vi "Main.vi"() -> ()   [LabVIEW 2018]
uses:
  Framework/CntrlRefs.ctl
  Modules/BusClass/Bus.lvclass/Bus.ctl
  LV_Config_class/Config.lvclass/Config.ctl
  Modules/Sync/SyncModule/PublicAPI/Arguments/Broadcasts/clDidInit.ctl
  <userlib>/NIST/ModuleAdminLib/ModuleAdmin/ModuleAdmin.lvclass
  LV_Config_class/Typedefs/eLogLvl.ctl
  Framework/UserEvents/clUserEventDataType.ctl
  LV_TestAutomation/Comms_lib/CommsData.ctl
  Modules/BusClass/Accessors/Read BusNumber.vi
  Modules/BusClass/Accessors/Read Test.vi
  LV_Config_class/Accessors/Read Root Directory.vi
  Modules/BusClass/Accessors/Write Test.vi
  LV_Config_class/Accessors/Read ConfigFilePath.vi
  <extravilib>/ChannelInstances/Tag-bool/Read With Abort.vi
  <extravilib>/ChannelInstances/Tag-bool/Write With Abort.vi
  <vilib>/Utility/error.llb/Error Cluster From Error Code.vi
  <extravilib>/ChannelInstances/Tag-bool/Instantiate.vi
  <extravilib>/ChannelInstances/Tag-bool/EndpointRead.vi
  <extravilib>/ChannelInstances/Tag-bool/Endpoint.vi
  <vilib>/ErrorRing/Error Ring.xnode
  Modules/TestClass/Test.lvclass
  Framework/Queue/Queue.lvlib
  <userlib>/NIST/NISTErrorLib/NISTErrorLib.lvlib
  LV_Config_class/Config.lvclass
  LV_Ini/Ini_lib.lvlib
  <vilib>/Utility/config.llb/NI_LVConfig.lvlib
  Modules/BusClass/Bus.lvclass
  Modules/Sync/SyncModule/SyncModule.lvlib
  Modules/FGen/FgenModule/FgenModule.lvlib
  Modules/Digitizer/DigitizerModule/DigitizerModule.lvlib
  Modules/Analysis/AnalysisModule/AnalysisModule.lvlib
  Modules/Sensor/SensorModule/SensorModule.lvlib
  Modules/Visualization/Visualization.lvlib
  LV_TestAutomation/LV-PY_Lib/LV-PY.lvlib
  LV_TestAutomation/Comms_lib/Comms.lvlib
  <extravilib>/ChannelInstances/Tag-bool.lvlib
panel:
  in  "btnAbort":bool
  in  "btnSettings":bool
  in  "btnHideMods":bool caption="Hide Modules"
  in  "chkLeaveScriptWindowOpen":bool
  in  "btnScriptFile":bool
  in  "Test Script":string
  in  "btnVisualize":bool
  out "Locked":bool
  in  "btnSyncPref":bool
  in  "rngSync":u16(ring) caption="Sync" items=["Local", "NI PXI 6682", "Debug Sync IOP", "6683H class Dyn3", "AbsPhase", "CorrFactor", "Debug", "SaveWaveform", "Dyn3 PMU Cal", "HIL_Sync", "INRM", "Legacy", "Offset Digi Trigger", "PXI Multi"]
  in  "btnSensorPref":bool
  in  "rngSensor":u16(ring) caption="Sensor" items=["C37.118 PMU", "C37.118 Sim", "Base PMU", "none", "Sim Ideal PMU"]
  in  "btnRunOne":bool
  in  "btnRunScript":bool
  in  "btnAnalysisPref":bool
  in  "rngAnalysis":u16(ring) caption="Analysis" items=["None", "AbsPhase", "FFT", "INRIM_Comp", "PMU", "AbsPhase_1M", "Analyse Waveforms"]
  in  "btnDigitizerPref":bool
  in  "rngDigitizer":u16(ring) caption="Digitizer" items=["Agilent3458", "IVI Digitizer", "AbsPhase_Current", "AbsPhase_Voltage", "Analyse Waveforms", "Debug", "INRiM_3Ch", "INRiM_4Ch", "INRiM_5Ch", "INRiM_6Ch", "INRM_1Ch", "Offset Trigger", "PMU Cal", "PRS_FGen", "Simulation"]
  in  "btnFGenPref":bool
  in  "rngFGen":u16(ring) caption="Function Generator" items=["DaqMx_Single", "Single_AM", "None", "Agilent IVI FGen", "IVI Dual FGens", "IVI FGen", "AbsPhase_Current_1Phase_ao3", "AbsPhase_Current_5A_ao0", "AbsPhase_Voltage_10V_Direct", "AbsPhase_Voltage_70V_Amp", "Debug", "INRM_1Ch", "INRM", "Pxi6733_Sine", "Pxi6733 Sine Standalone", "PMU Cal", "PMU_Sim", "Test"]
  in  "btnTestFile":bool
  in  "Test File":string
  in  "btnStop":bool
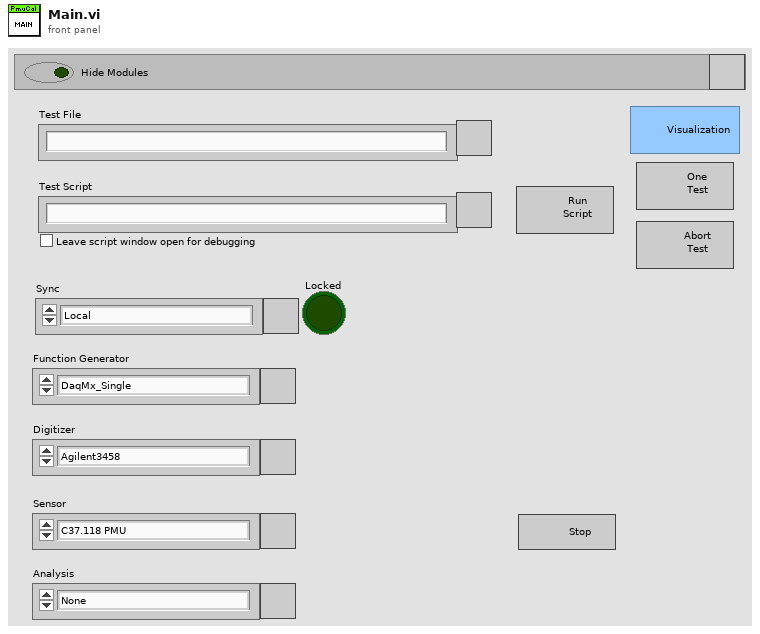
[diagram p1: front panel]
types:
  T1 = typedef "CntrlRefs.ctl" = cluster{"rngFGen":refnum<vi>, "rngDigitizer":refnum<vi>, "rngAnalysis":refnum<vi>, "rngSync":refnum<vi>, "btnHideMods":refnum<vi>, "rngSensor":refnum<vi>, "Test Script":refnum<vi>}
  T2 = typedef "SyncModule.lvlib/clBroadcastEvents.ctl" = cluster{"DidInit":refnum<user-event>, "StatusUpdate":refnum<user-event>, "ErrorReport":refnum<user-event>, "DidStop":refnum<user-event>, "PathToINI":refnum<user-event>, "TriggerTime":refnum<user-event>, "LockStatus":refnum<user-event>, "Info":refnum<user-event>, "ClockProperties":refnum<user-event>}
  T3 = typedef "FgenModule.lvlib/clBroadcastEvents.ctl" = cluster{"DidInit":refnum<user-event>, "StatusUpdate":refnum<user-event>, "ErrorReport":refnum<user-event>, "DidStop":refnum<user-event>, "PathToINI":refnum<user-event>, "Channels":refnum<user-event>, "Function":refnum<user-event>, "Waveforms":refnum<user-event>, "Triggers":refnum<user-event>, "FunctionParams":refnum<user-event>, "FunctionArbs":refnum<user-event>, "FunctionSampleRate":refnum<user-event>}
  T4 = typedef "DigitizerModule.lvlib/clBroadcastEvents.ctl" = cluster{"DidInit":refnum<user-event>, "StatusUpdate":refnum<user-event>, "ErrorReport":refnum<user-event>, "DidStop":refnum<user-event>, "PathToINI":refnum<user-event>, "Channels":refnum<user-event>, "Acq":refnum<user-event>, "Trigger":refnum<user-event>, "Waveforms":refnum<user-event>}
  T5 = typedef "SensorShared.lvlib/clBroadcastEvents.ctl" = cluster{"DidInit":refnum<user-event>, "StatusUpdate":refnum<user-event>, "ErrorReport":refnum<user-event>, "DidStop":refnum<user-event>, "PathToINI":refnum<user-event>, "SensorReport":refnum<user-event>, "SensorConfig":refnum<user-event>}
  T6 = typedef "AnalysisModule.lvlib/clBroadcastEvents.ctl" = cluster{"DidInit":refnum<user-event>, "StatusUpdate":refnum<user-event>, "ErrorReport":refnum<user-event>, "DidStop":refnum<user-event>, "PathToINI":refnum<user-event>, "Config":refnum<user-event>, "ResultReport":refnum<user-event>, "FunctionClass":refnum<user-event>, "State":refnum<user-event>, "FunctionParams":refnum<user-event>}
  T7 = typedef "clUserEvents.ctl" = cluster{"StopEvent":refnum<user-event>, "CreateBus":refnum<user-event>, "UpdateEvents":refnum<user-event>}
  T8 = typedef "clUserEventDataType.ctl" = cluster{"Data":variant}
  T9 = typedef "Comms.lvlib/CommsData.ctl" = cluster{"Command":string, "XMLData":string}
  T10 = typedef "NI_LVConfig.lvlib/Config Data RefNum.ctl" = refnum<k1>
  T11 = typedef "Config_class.lvlib/Config.lvclass/RootDir.ctl" = cluster{"pathRootDir":path, "btnOutPath":bool, "OutDir":string, "btnOpenOutputDir":bool, "ScriptDir":string, "btnOpenScriptDir":bool, "TestDir":string, "btnOpenTestDir":bool}
  T12 = typedef "Tag-bool.lvlib/))Channel.ctl" = refnum<queue>
  T13 = typedef "Config_class.lvlib/Config.lvclass/eLogLvl.ctl" = enum16{"Normal", "Verbose", "None"}
  T14 = typedef "SyncModule.lvlib/clDidInit.ctl" = cluster{"Init?":bool, "ModuleAdmin":refnum<class "ModuleAdmin.lvclass">}
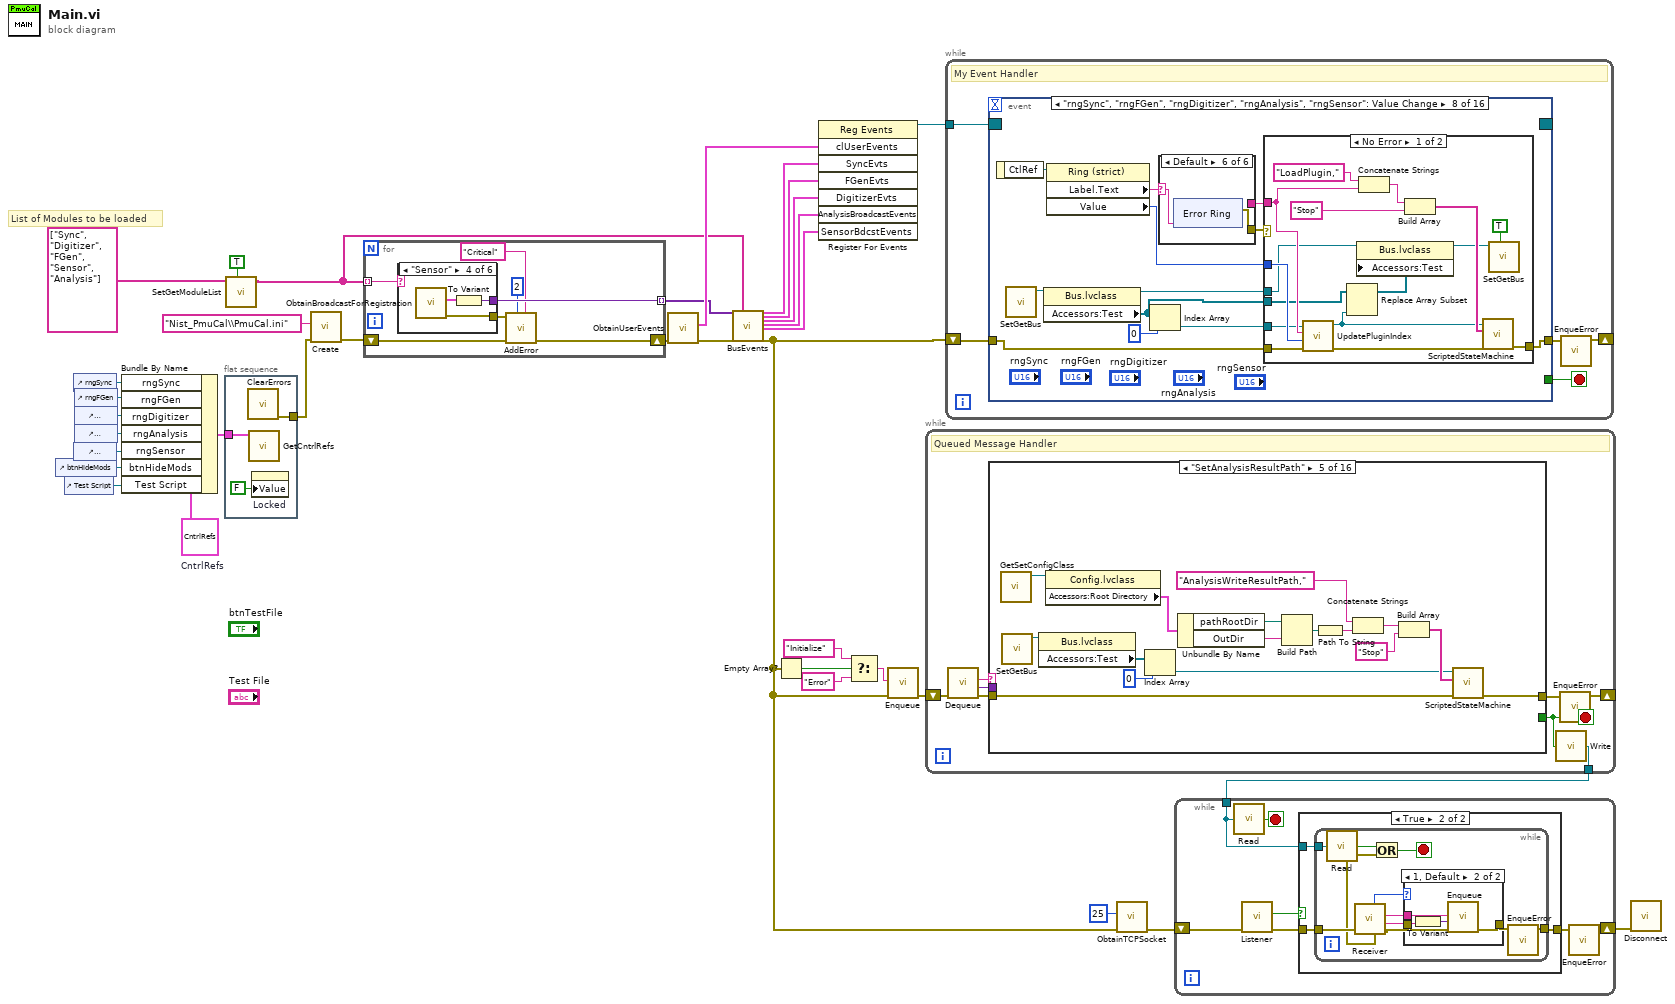
[diagram p0: block diagram]
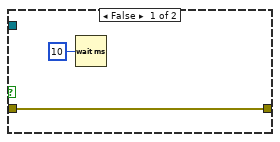
[diagram p2: hidden frame]
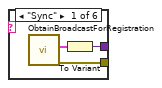
[diagram p4: hidden frame]
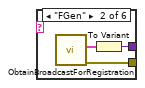
[diagram p5: hidden frame]
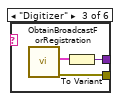
[diagram p6: hidden frame]
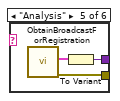
[diagram p7: hidden frame]
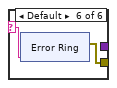
[diagram p8: hidden frame]
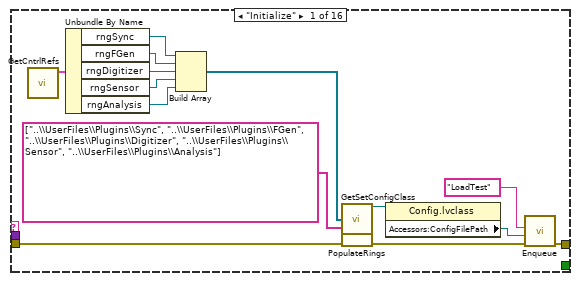
[diagram p9: hidden frame]
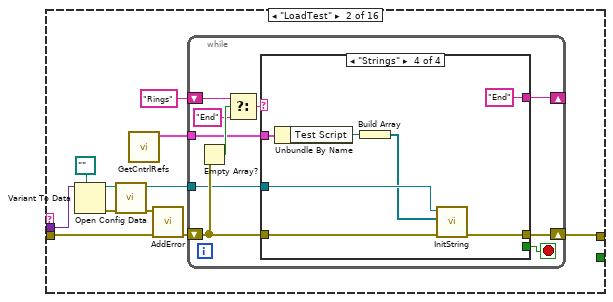
[diagram p10: hidden frame]
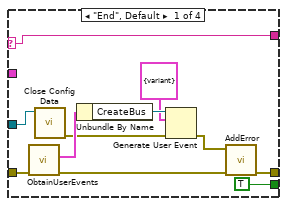
[diagram p11: hidden frame]
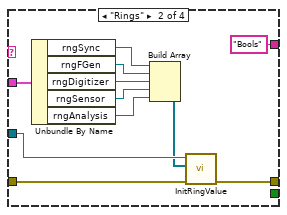
[diagram p12: hidden frame]
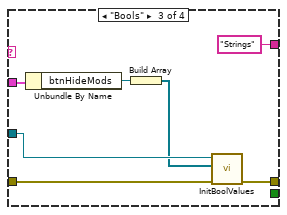
[diagram p13: hidden frame]
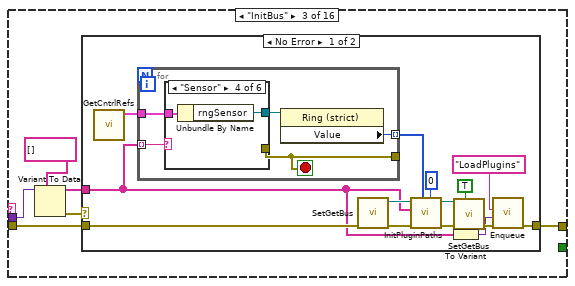
[diagram p14: hidden frame]
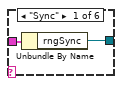
[diagram p15: hidden frame]
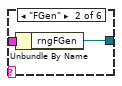
[diagram p16: hidden frame]
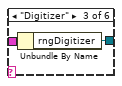
[diagram p17: hidden frame]
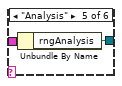
[diagram p18: hidden frame]
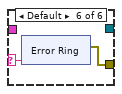
[diagram p19: hidden frame]
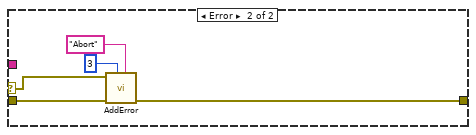
[diagram p20: hidden frame]
diagram:
  w31 = T1 {"rngFGen"=refnum, "rngDigitizer"=refnum, "rngAnalysis"=refnum, "rngSync"=refnum, "btnHideMods"=refnum, "rngSensor"=refnum, "Test Script"=refnum}  # CntrlRefs
  # "List of Modules to be loaded"
  n1 = control-ref of="btnHideMods"() -> (w9:refnum<vi>)
  n2 = control-ref of="Test Script"() -> (w2:refnum<vi>)
  n3 = control-ref of="rngSync"() -> (w23:refnum<vi>)
  n4 = control-ref of="rngSensor"() -> (w8:refnum<vi>)
  n5 = control-ref of="rngFGen"() -> (w30:refnum<vi>)
  n6 = control-ref of="rngDigitizer"() -> (w28:refnum<vi>)
  n7 = control-ref of="rngAnalysis"() -> (w27:refnum<vi>)
  n8 = Bundle By Name(cluster=w31, "rngSync"=w23, "rngFGen"=w30, "rngDigitizer"=w28, "rngAnalysis"=w27, "rngSensor"=w8, "btnHideMods"=w9, "Test Script"=w2) -> (w29:T1)
  n9 = flat-sequence {
    tunnel: [w38] -> w32
    tunnel: w29 -> [w37]
    frame #0 {
      n10 = call <userlib>:"ClearErrors.vi"() -> ("ErrorArray"=w38:errorcluster[])  [unwired: 11 in]
      n11 = call "GetCntrlRefs.vi"("CntrlRefs"=w37) -> ()  [unwired: 10 in, 1 out]
      n12 = property on="Locked" class="Bool (strict)"("Value"=FALSE) -> ()  [unwired: 2 in, 2 out]
    }
  }
  n13 = call "SetGetModuleList.vi"("Set? (f)"=TRUE, "ModuleList"=string[] ["Sync", "Digitizer", "FGen", "Sensor", "Analysis"]) -> ("ModuleList"=w12:string[])  [unwired: 9 in]
  n14 = call "Create.vi"("ErrorArray"=w32, "name or relative path"="Nist_PmuCal\\PmuCal.ini") -> ("ErrorArray"=w18:errorcluster[])  [unwired: 8 in, 1 out]
  n15 = for {
    shift-right: [w44] -> w17
    shift-left: w18 -> [w43]
    tunnel: [w42] -> w14 mode=indexing
    tunnel: w12 -> [w39] mode=indexing
    n16 = case shown="\"Sensor\"" w39 {
      selector: w39 -> [_ _ _ _ _ w61]
      tunnel: [w47 w50 w53 w56 w59 _] -> w42
      tunnel: [w46 w51 w54 w57 w60 w62] -> w45
      frame "Sync" {
        n17 = call "ObtainBroadcastForRegistration.vi"() -> ("error out"=w46:errorcluster, "SyncBroadcastEvents"=w48:T2)  [unwired: 10 in]
        n18 = To Variant(anything=w48) -> (Variant=w47:variant)
      }
      frame "FGen" {
        n19 = call "ObtainBroadcastForRegistration.vi"() -> ("error out"=w51:errorcluster, "clBroadcastEvents"=w49:T3)  [unwired: 10 in]
        n20 = To Variant(anything=w49) -> (Variant=w50:variant)
      }
      frame "Digitizer" {
        n21 = call "ObtainBroadcastForRegistration.vi"() -> ("error out"=w54:errorcluster, "clDigitizerBdcstEvents"=w52:T4)  [unwired: 10 in]
        n22 = To Variant(anything=w52) -> (Variant=w53:variant)
      }
      frame "Sensor" {
        n23 = call "ObtainBroadcastForRegistration.vi"() -> ("error out"=w57:errorcluster, "SensorBdcstEvents"=w55:T5)  [unwired: 10 in]
        n24 = To Variant(anything=w55) -> (Variant=w56:variant)
      }
      frame "Analysis" {
        n25 = call "ObtainBroadcastForRegistration.vi"() -> ("error out"=w60:errorcluster, "AnalysisBroadcastEvents"=w58:T6)  [unwired: 10 in]
        n26 = To Variant(anything=w58) -> (Variant=w59:variant)
      }
      frame Default {
        n27 = xnode "Error Ring"("parameter 0"=w61) -> ("error out"=w62:errorcluster)
      }
    }
    n28 = call <userlib>:"AddError.vi"("Severity"="Critical", "Priority"=u8 2, "ErrorArray"=w43, "error in (no error)"=w45) -> ("ErrorArray"=w44:errorcluster[])  [unwired: 6 in, 1 out]
  }
  n29 = call "ObtainUserEvents.vi"("ErrorArray"=w17) -> ("ErrorArray"=w16:errorcluster[], "clUserEvents"=w15:T7)  [unwired: 9 in]
  n30 = call "BusEvents.vi"("EventArray"=w14, "Error in"=w16, "ModuleList"=w12) -> ("SyncEvts"=w26:T2, "FGenEvts"=w25:T3, "DigitizerEvts"=w24:T4, "AnalysisBroadcastEvents"=w10:T6, "SensorBdcstEvents"=w7:T5, "Error out"=w6:errorcluster[])  [unwired: 16 in, 3 out]
  n31 = Empty Array?(array=w6) -> (empty?=w22:bool)
  n32 = register-events(w15, w26, w25, w24, w10, w7) -> (reference out=w35:refnum<event-registration>)  [unwired: 2 in, 1 out]
  n33 = Select(t="Initialize" ("Message"), s=w22, f="Error" ("Message")) -> (s? t:f=w19:string)
  n34 = call "Enqueue.vi"("ErrorArray"=w6, "Message"=w19) -> ("ErrorArray"=w34:errorcluster[])  [unwired: 9 in]
  n35 = while {
    shift-right: [w74] -> _
    shift-left: w34 -> [w77]
    tunnel: [w70] -> w1
    stop <- w71 stop-if-true
    # "Queued Message Handler"
    n36 = call "Dequeue.vi"("ErrorArray"=w77) -> ("ErrorArray"=w73:errorcluster[], "Message Data"=w72:variant, "Message"=w76:string)  [unwired: 8 in]
    n37 = case shown="\"SetAnalysisResultPath\"" w76 {
      selector: w76 -> [_ _ _ _ _ _ _ _ _ _ _ _ _ _ _ w415]
      tunnel: [w90 w93 w151 w198 w222 w240 w296 w306 w329 w349 w356 w366 w372 w375 w388 w413] -> w75
      tunnel: w73 -> [w86 w98 w152 w199 w228 w246 w301 w320 w333 w353 w360 w367 w374 w376 _ w412]
      tunnel: [_ _ _ _ _ _ _ _ _ _ _ _ _ TRUE _ _] -> w71
      tunnel: w72 -> [_ w97 w154 w201 _ w248 _ _ w335 w355 w364 _ _ _ w392 _]
      frame "Initialize" {
        n38 = call "GetCntrlRefs.vi"() -> ("CntrlRefs"=w85:T1)  [unwired: 11 in]
        n39 = Unbundle By Name(w85) -> ("rngSync"=w79:refnum<vi>, "rngFGen"=w84:refnum<vi>, "rngDigitizer"=w83:refnum<vi>, "rngSensor"=w82:refnum<vi>, "rngAnalysis"=w78:refnum<vi>)
        n40 = Build Array(w79, w84, w83, w82, w78) -> (w80:refnum<vi>[])
        n41 = call "GetSetConfigClass.vi"() -> ("Ref out"=w91:refnum<class "Config.lvclass">)  [unwired: 11 in]
        n42 = call "PopulateRings.vi"("ErrorArray In"=w86, "RelativePathToIniArray"=string[] ["..\\UserFiles\\Plugins\\Sync", "..\\UserFiles\\Plugins\\FGen", "..\\UserFiles\\Plugins\\Digitizer", "..\\UserFiles\\Plugins\\Sensor", "..\\UserFiles\\Plugins\\Analysis"], "RingRefArray"=w80) -> ("ErrorArray Out"=w87:errorcluster[])  [unwired: 7 in, 1 out]
        n43 = property class="Config.lvclass"(reference=w91) -> ("Accessors:ConfigFilePath"=w89:path)  [unwired: 1 in, 2 out]
        n44 = call "Enqueue.vi"("ErrorArray"=w87, "Message Data"=w89, "Message"="LoadTest") -> ("ErrorArray"=w90:errorcluster[])  [unwired: 8 in]
      }
      frame "LoadTest" {
        n45 = Variant To Data(type=path "", Variant=w97) -> (data=w101:path, error out=w99:errorcluster)  [unwired: 1 in]
        n46 = call <vilib>:"Open Config Data.vi"("error in (no error)"=w99, "configuration file path"=w101) -> ("error out"=w100:errorcluster, "refnum"=w95:T10)  [unwired: 7 in, 1 out]
        n47 = call "GetCntrlRefs.vi"() -> ("CntrlRefs"=w92:T1)  [unwired: 11 in]
        n48 = call <userlib>:"AddError.vi"("ErrorArray"=w98, "error in (no error)"=w100) -> ("ErrorArray"=w96:errorcluster[])  [unwired: 8 in, 1 out]
        n49 = while {
          shift-right: [w106] -> w93
          shift-left: w96 -> [w108]
          tunnel: w95 -> [w107]
          shift-right: [w104] -> _
          shift-left: "Rings" -> [w111]
          tunnel: w92 -> [w103]
          stop <- w105 stop-if-true
          n50 = Empty Array?(array=w108) -> (empty?=w112:bool)
          n51 = Select(t=w111, s=w112, f="End") -> (s? t:f=w109:string)
          n52 = case shown="\"Strings\"" w109 {
            selector: w109 -> [w120 _ _ _]
            tunnel: w108 -> [w119 w134 w139 w147]
            tunnel: w107 -> [w123 w133 w137 w145]
            tunnel: [w122 w127 w138 w146] -> w106
            tunnel: [TRUE _ _ _] -> w105
            tunnel: [w120 "Bools" "Strings" "End"] -> w104
            tunnel: w103 -> [_ w126 w140 w144]
            frame "End", Default {
              n53 = call "ObtainUserEvents.vi"("ErrorArray"=w119) -> ("ErrorArray"=w113:errorcluster[], "clUserEvents"=w118:T7)  [unwired: 9 in]
              n54 = call <vilib>:"Close Config Data.vi"("refnum"=w123) -> ("error out"=w116:errorcluster)  [unwired: 9 in, 1 out]
              n55 = Unbundle By Name(w118) -> ("CreateBus"=w117:refnum<user-event>)
              n56 = Generate User Event(user event=w117, event data cluster=T8 {"Data"=variant} ("clUserEventData"), error in=w116) -> (error out=w114:errorcluster)  [unwired: 1 in, 1 out]
              n57 = call <userlib>:"AddError.vi"("ErrorArray"=w113, "error in (no error)"=w114) -> ("ErrorArray"=w122:errorcluster[])  [unwired: 8 in, 1 out]
            }
            frame "Rings" {
              n58 = Unbundle By Name(w126) -> ("rngSync"=w125:refnum<vi>, "rngFGen"=w130:refnum<vi>, "rngDigitizer"=w131:refnum<vi>, "rngSensor"=w129:refnum<vi>, "rngAnalysis"=w124:refnum<vi>)
              n59 = Build Array(w125, w130, w131, w129, w124) -> (w128:refnum<vi>[])
              n60 = call "InitRingValue.vi"("ErrorArray In"=w134, "RingRefArray"=w128, "IniFileRef"=w133) -> ("ErrorArray Out"=w127:errorcluster[])  [unwired: 6 in, 2 out]
            }
            frame "Bools" {
              n61 = Unbundle By Name(w140) -> ("btnHideMods"=w136:refnum<vi>)
              n62 = Build Array(w136) -> (w135:refnum<vi>[])
              n63 = call "InitBoolValues.vi"("ErrorArray in"=w139, "BoolRefArray"=w135, "IniFileRef in"=w137) -> ("ErrorArray Out"=w138:errorcluster[])  [unwired: 7 in, 1 out]
            }
            frame "Strings" {
              n64 = Unbundle By Name(w144) -> ("Test Script"=w143:refnum<vi>)
              n65 = Build Array(w143) -> (w142:refnum<vi>[])
              n66 = call "InitString.vi"("ErrorArray in"=w147, "StringRefArray"=w142, "IniFileRef in"=w145) -> ("ErrorArray Out"=w146:errorcluster[])  [unwired: 7 in, 1 out]
            }
          }
        }
      }
      frame "InitBus" {
        n67 = Variant To Data(type=string[] [], Variant=w154) -> (data=w150:string[], error out=w149:errorcluster)  [unwired: 1 in]
        n68 = case shown="No Error" w149 {
          selector: w149 -> [_ w193]
          tunnel: w152 -> [w166 w195]
          tunnel: [w158 w194] -> w151
          tunnel: w150 -> [w155 _]
          frame No Error {
            n69 = call "GetCntrlRefs.vi"() -> ("CntrlRefs"=w165:T1)  [unwired: 11 in]
            n70 = for {
              tunnel: w155 -> [w171] mode=indexing
              tunnel: w165 -> [w170]
              tunnel: [w168] -> w163 mode=indexing
              tunnel: [w167] -> _
              stop <- w167 stop-if-true
              n71 = case shown="\"Sensor\"" w171 {
                selector: w171 -> [_ _ _ _ _ w183]
                tunnel: w170 -> [w173 w175 w177 w179 w181 _]
                tunnel: [w172 w174 w176 w178 w180 _] -> w169
                tunnel: [_ _ _ _ _ w182] -> w167
                frame "Sync" {
                  n72 = Unbundle By Name(w173) -> ("rngSync"=w172:refnum<vi>)
                }
                frame "FGen" {
                  n73 = Unbundle By Name(w175) -> ("rngFGen"=w174:refnum<vi>)
                }
                frame "Digitizer" {
                  n74 = Unbundle By Name(w177) -> ("rngDigitizer"=w176:refnum<vi>)
                }
                frame "Sensor" {
                  n75 = Unbundle By Name(w179) -> ("rngSensor"=w178:refnum<vi>)
                }
                frame "Analysis" {
                  n76 = Unbundle By Name(w181) -> ("rngAnalysis"=w180:refnum<vi>)
                }
                frame Default {
                  n77 = xnode "Error Ring"("parameter 0"=w183) -> ("error out"=w182:errorcluster)
                }
              }
              n78 = property class="Ring (strict)"(reference=w169) -> ("Value"=w168:u16)  [unwired: 1 in, 2 out]
            }
            n79 = call "SetGetBus.vi"() -> ("Bus.lvclass"=w164:refnum<class "Bus.lvclass">)  [unwired: 11 in]
            n80 = call "InitPluginPaths.vi"("BusIndex"=0, "PluginIndex"=w163, "Error In"=w166, "Modules"=w155, "Bus in"=w164) -> ("Error Out"=w159:errorcluster[], "Bus out"=w161:refnum<class "Bus.lvclass">)  [unwired: 5 in]
            n81 = To Variant(anything=w155) -> (Variant=w156:variant)
            n82 = call "SetGetBus.vi"("Set (f)"=TRUE, "Bus.lvclass"=w161) -> ()  [unwired: 9 in, 1 out]
            n83 = call "Enqueue.vi"("ErrorArray"=w159, "Message Data"=w156, "Message"="LoadPlugins") -> ("ErrorArray"=w158:errorcluster[])  [unwired: 8 in]
          }
          frame Error {
            n84 = call <userlib>:"AddError.vi"("Severity"="Abort", "Priority"=u8 3, "ErrorArray"=w195, "error in (no error)"=w193) -> ("ErrorArray"=w194:errorcluster[])  [unwired: 6 in, 1 out]
          }
        }
      }
      frame "LoadPlugins" {
        n85 = Variant To Data(type=string[] [], Variant=w201) -> (data=w197:string[], error out=w196:errorcluster)  [unwired: 1 in]
        n86 = case shown="No Error" w196 {
          selector: w196 -> [_ w219]
          tunnel: w199 -> [w210 w221]
          tunnel: [w203 w220] -> w198
          tunnel: w197 -> [w213 _]
          frame No Error {
            n87 = for {
              tunnel: w213 -> [w215] mode=indexing
              tunnel: [w214] -> w212 mode=indexing
              n88 = Concatenate Strings("LoadPlugin," ("string"), w215) -> (w214:string)
            }
            n89 = call "SetGetBus.vi"() -> ("Bus.lvclass"=w209:refnum<class "Bus.lvclass">)  [unwired: 11 in]
            n90 = property class="Bus.lvclass"(reference=w209) -> ("Accessors:Test"=w208:refnum<class "Test.lvclass">[])  [unwired: 1 in, 2 out]
            n91 = Index Array(array=w208, index=0) -> (element=w206:refnum<class "Test.lvclass">)
            n92 = Build Array (concatenate)(w212, "Stop" ("string")) -> (w205:string[])
            n93 = call "ScriptedStateMachine.vi"("ErrorArray"=w210, "script"=w205, "Test.lvclass"=w206) -> ("ErrorArray"=w204:errorcluster[])  [unwired: 6 in, 2 out]
            n94 = call "Enqueue.vi"("ErrorArray"=w204, "Message"="SetAnalysisResultPath") -> ("ErrorArray"=w203:errorcluster[])  [unwired: 9 in]
          }
          frame Error {
            n95 = call <userlib>:"AddError.vi"("Severity"="Abort", "Priority"=u8 3, "ErrorArray"=w221, "error in (no error)"=w219) -> ("ErrorArray"=w220:errorcluster[])  [unwired: 6 in, 1 out]
          }
        }
      }
      frame "SetAnalysisResultPath" {
        n96 = call "GetSetConfigClass.vi"() -> ("Ref out"=w237:refnum<class "Config.lvclass">)  [unwired: 11 in]
        n97 = call "SetGetBus.vi"() -> ("Bus.lvclass"=w226:refnum<class "Bus.lvclass">)  [unwired: 11 in]
        n98 = property class="Bus.lvclass"(reference=w226) -> ("Accessors:Test"=w225:refnum<class "Test.lvclass">[])  [unwired: 1 in, 2 out]
        n99 = property class="Config.lvclass"(reference=w237) -> ("Accessors:Root Directory"=w236:T11)  [unwired: 1 in, 2 out]
        n100 = Index Array(array=w225, index=0) -> (element=w223:refnum<class "Test.lvclass">)
        n101 = Unbundle By Name(w236) -> ("pathRootDir"=w235:path, "OutDir"=w234:string)
        n102 = Build Path(base path=w235, name or relative path=w234) -> (appended path=w233:path)
        n103 = Path To String(path=w233) -> (string=w232:string)
        n104 = Concatenate Strings("AnalysisWriteResultPath,", w232) -> (w230:string)
        n105 = Build Array(w230, "Stop") -> (w227:string[])
        n106 = call "ScriptedStateMachine.vi"("ErrorArray"=w228, "script"=w227, "Test.lvclass"=w223) -> ("ErrorArray"=w222:errorcluster[])  [unwired: 6 in, 2 out]
      }
      frame "SaveTest" {
        n107 = Variant To Data(type=path "", Variant=w248) -> (data=w244:path, error out=w239:errorcluster)  [unwired: 1 in]
        n108 = call <vilib>:"Open Config Data.vi"("error in (no error)"=w239, "configuration file path"=w244) -> ("error out"=w243:errorcluster, "refnum"=w242:T10)  [unwired: 7 in, 1 out]
        n109 = call "GetCntrlRefs.vi"() -> ("CntrlRefs"=w238:T1)  [unwired: 11 in]
        n110 = call <userlib>:"AddError.vi"("ErrorArray"=w246, "error in (no error)"=w243) -> ("ErrorArray"=w245:errorcluster[])  [unwired: 8 in, 1 out]
        n111 = while {
          tunnel: w242 -> [w258]
          shift-right: [w252] -> w240
          shift-left: w245 -> [w254]
          shift-right: [w250] -> _
          shift-left: "Rings" -> [w256]
          tunnel: w238 -> [w249]
          stop <- w251 stop-if-true
          n112 = Empty Array?(array=w254) -> (empty?=w255:bool)
          n113 = Select(t=w256, s=w255, f="end") -> (s? t:f=w257:string)
          n114 = case shown="\"Bools\"" w257 {
            selector: w257 -> [_ _ _ w284]
            tunnel: w254 -> [w266 w273 w283 w286]
            tunnel: w258 -> [w265 w272 w281 w289]
            tunnel: [w263 w270 w282 w285] -> w252
            tunnel: [_ _ _ TRUE] -> w251
            tunnel: ["Bools" "Strings" "End" w284] -> w250
            tunnel: w249 -> [w260 w275 w280 _]
            frame "Rings" {
              n115 = Unbundle By Name(w260) -> ("rngSync"=w261:refnum<vi>, "rngFGen"=w267:refnum<vi>, "rngDigitizer"=w269:refnum<vi>, "rngSensor"=w268:refnum<vi>, "rngAnalysis"=w259:refnum<vi>)
              n116 = Build Array(w261, w267, w269, w268, w259) -> (w264:refnum<vi>[])
              n117 = call "RingsToIni.vi"("ErrorArray in"=w266, "RingRefArray"=w264, "IniFileRef in"=w265) -> ("ErrorArray out"=w263:errorcluster[])  [unwired: 7 in, 1 out]
            }
            frame "Bools" {
              n118 = Unbundle By Name(w275) -> ("btnHideMods"=w274:refnum<vi>)
              n119 = Build Array(w274) -> (w271:refnum<vi>[])
              n120 = call "BoolsToIni.vi"("ErrorArray in"=w273, "BoolRefArray"=w271, "IniFileRef in"=w272) -> ("ErrorArray out"=w270:errorcluster[])  [unwired: 7 in, 1 out]
            }
            frame "Strings" {
              n121 = Unbundle By Name(w280) -> ("Test Script"=w279:refnum<vi>)
              n122 = Build Array(w279) -> (w278:refnum<vi>[])
              n123 = call "StringToIni.vi"("ErrorArray in"=w283, "StringRefArray"=w278, "IniFileRef in"=w281) -> ("ErrorArray out"=w282:errorcluster[])  [unwired: 7 in, 1 out]
            }
            frame "End", Default {
              n124 = call <vilib>:"Close Config Data.vi"("write file if changed (T)"=TRUE, "refnum"=w289) -> ("error out"=w287:errorcluster)  [unwired: 8 in, 1 out]
              n125 = call <userlib>:"AddError.vi"("ErrorArray"=w286, "error in (no error)"=w287) -> ("ErrorArray"=w285:errorcluster[])  [unwired: 8 in, 1 out]
            }
          }
        }
      }
      frame "RunOneTest" {
        n126 = call "SetGetModuleList.vi"() -> ("ModuleList"=w293:string[])  [unwired: 11 in]
        n127 = call "SetGetBus.vi"() -> ("Bus.lvclass"=w300:refnum<class "Bus.lvclass">)  [unwired: 11 in]
        n128 = for {
          tunnel: w293 -> [w303] mode=indexing
          shift-right: [w302] -> w294
          shift-left: "RunTest" -> [w305]
          n129 = Concatenate Strings(w305, ",", w303) -> (w302:string)
        }
        n130 = property class="Bus.lvclass"(reference=w300) -> ("Accessors:Test"=w299:refnum<class "Test.lvclass">[])  [unwired: 1 in, 2 out]
        n131 = Index Array(array=w299, index=0) -> (element=w297:refnum<class "Test.lvclass">)
        n132 = Build Array(w294, "Stop") -> (w292:string[])
        n133 = call "ScriptedStateMachine.vi"("ErrorArray"=w301, "script"=w292, "Test.lvclass"=w297) -> ("ErrorArray"=w296:errorcluster[])  [unwired: 6 in, 2 out]
      }
      frame "run" {
        # "TODO: figure out how to send SSM errors to Python"
        n134 = call "SetGetBus.vi"() -> ("Bus.lvclass"=w319:refnum<class "Bus.lvclass">)  [unwired: 11 in]
        n135 = call "SetGetModuleList.vi"() -> ("ModuleList"=w313:string[])  [unwired: 11 in]
        n136 = property class="Bus.lvclass"(reference=w319) -> ("Accessors:Test"=w318:refnum<class "Test.lvclass">[])  [unwired: 1 in, 2 out]
        n137 = for {
          tunnel: w313 -> [w322] mode=indexing
          shift-right: [w321] -> w314
          shift-left: "RunTest" -> [w324]
          n138 = Concatenate Strings(w324, ",", w322) -> (w321:string)
        }
        n139 = Index Array(array=w318, index=0) -> (element=w316:refnum<class "Test.lvclass">)
        n140 = Build Array(w314, "Stop") -> (w312:string[])
        n141 = call "ScriptedStateMachine.vi"("ErrorArray"=w320, "script"=w312, "Test.lvclass"=w316) -> ("ErrorArray"=w309:errorcluster[])  [unwired: 6 in, 2 out]
        n142 = Flatten To XML(anything=errorcluster {"status"=FALSE, "code"=0, "source"=""} ("error constant")) -> (xml string=w308:string)
        n143 = call "Transmitter.vi"("ErrorArray"=w309, "XMLData"=w308, "Command"="LtaRunComplete") -> ("ErrorArray"=w306:errorcluster[])  [unwired: 7 in, 1 out]
      }
      frame "get" {
        n144 = Variant To Data(type="", Variant=w335) -> (data=w330:string, error out=w332:errorcluster)  [unwired: 1 in]
        n145 = call "SetGetBus.vi"() -> ("Bus.lvclass"=w328:refnum<class "Bus.lvclass">)  [unwired: 11 in]
        n146 = property class="Bus.lvclass"(reference=w328) -> ("Accessors:Test"=w327:refnum<class "Test.lvclass">[])  [unwired: 1 in, 2 out]
        n147 = call <userlib>:"AddError.vi"("ErrorArray"=w333, "error in (no error)"=w332) -> ("ErrorArray"=w331:errorcluster[])  [unwired: 8 in, 1 out]
        n148 = Index Array(array=w327, index=0) -> (element=w326:refnum<class "Test.lvclass">)
        n149 = call "LtaGetModuleProperties.vi"("Error In"=w331, "arg"=w330, "Test.lvclass"=w326) -> ("Error Out"=w329:errorcluster[])  [unwired: 6 in, 2 out]
      }
      frame "set" {
        n150 = call "SetGetBus.vi"() -> ("Bus.lvclass"=w339:refnum<class "Bus.lvclass">)  [unwired: 11 in]
        n151 = Variant To Data(type="", Variant=w355) -> (data=w345:string, error out=w344:errorcluster)  [unwired: 1 in]
        n152 = property class="Bus.lvclass"(reference=w339) -> ("Accessors:Test"=w338:refnum<class "Test.lvclass">[])  [unwired: 1 in, 2 out]
        n153 = Unflatten From XML(xml string=w345, type=T9 {"Command"="", "XMLData"=""} ("CommsData"), error in (no error)=w344) -> (value=w342:T9, error out=w343:errorcluster)
        n154 = call <userlib>:"AddError.vi"("ErrorArray"=w353, "error in (no error)"=w343) -> ("ErrorArray"=w348:errorcluster[])  [unwired: 8 in, 1 out]
        n155 = Unbundle By Name(w342) -> ("Command"=w340:string, "XMLData"=w341:string)
        n156 = Index Array(array=w338, index=0) -> (element=w337:refnum<class "Test.lvclass">)
        n157 = call "LtaSetModuleProperties.vi"("Error In"=w348, "XmlData"=w341, "Arg"=w340, "Test.lvclass"=w337) -> ("Error Out"=w347:errorcluster[])  [unwired: 6 in, 1 out]
        n158 = Flatten To XML(anything=errorcluster {"status"=FALSE, "code"=0, "source"=""} ("error constant")) -> (xml string=w350:string)
        n159 = call "Transmitter.vi"("ErrorArray"=w347, "XMLData"=w350, "Command"="LtaSetComplete") -> ("ErrorArray"=w349:errorcluster[])  [unwired: 7 in, 1 out]
      }
      frame "ClientError" {
        n160 = Variant To Data(type="", Variant=w364) -> (data=w362:string, error out=w361:errorcluster)  [unwired: 1 in]
        n161 = Unflatten From XML(xml string=w362, type=w361, error in (no error)=w361) -> (value=w357:errorcluster, error out=w359:errorcluster)
        n162 = call <userlib>:"AddError.vi"("ErrorArray"=w360, "error in (no error)"=w359) -> ("ErrorArray"=w358:errorcluster[])  [unwired: 8 in, 1 out]
        n163 = Build Array (concatenate)(w358, w357) -> (w356:errorcluster[])
      }
      frame "Visualize" {
        n164 = call "dlgSelectVisApps.vi"("Error In"=w367, "PathsToVisApps"=string[] ["VisualizeStatus", "VisualizeAnalysis", "VisualizeDigitizer"]) -> ("Error Out"=w366:errorcluster[])  [unwired: 9 in]
      }
      frame "Stop" {
        n165 = call "GetSetConfigClass.vi"() -> ("Ref out"=w370:refnum<class "Config.lvclass">)  [unwired: 11 in]
        n166 = property class="Config.lvclass"(reference=w370) -> ("Accessors:ConfigFilePath"=w369:path)  [unwired: 1 in, 2 out]
        n167 = call "Enqueue.vi"("ErrorArray"=w374, "Message Data"=w369, "Message"="SaveTest") -> ("ErrorArray"=w373:errorcluster[])  [unwired: 8 in]
        n168 = call "Enqueue.vi"("ErrorArray"=w373, "Message"="End") -> ("ErrorArray"=w372:errorcluster[])  [unwired: 9 in]
      }
      frame "End" {
        n169 = call "SetGetBus.vi"() -> ("Bus.lvclass"=w379:refnum<class "Bus.lvclass">)  [unwired: 11 in]
        n170 = property class="Bus.lvclass"(reference=w379) -> (reference out=w381:refnum<class "Bus.lvclass">, "Accessors:BusNumber"=w380:i32[])  [unwired: 1 in, 1 out]
        n171 = for {
          tunnel: w380 -> [w384] mode=indexing
          shift-right: [w385] -> w375
          shift-left: w376 -> [w386]
          shift-right: [w383] -> w378
          shift-left: w381 -> [w387]
          n172 = call "RemoveBus.vi"("BusNumber"=w384, "ErrorIn"=w386, "Bus.lvclass"=w387) -> ("ErrorOut"=w385:errorcluster[], "Bus.lvclass"=w383:refnum<class "Bus.lvclass">)  [unwired: 7 in]
        }
        n173 = call "SetGetBus.vi"("Set (f)"=TRUE, "Bus.lvclass"=w378) -> ()  [unwired: 9 in, 1 out]
      }
      frame "Error" {
        n174 = Variant To Data(type=errorcluster[] [] ("ErrorArray"), Variant=w392) -> (data=w390:errorcluster[])  [unwired: 1 in, 1 out]
        n175 = call <userlib>:"ParseErrors.vi"("ErrorArray"=w390) -> ("ErrorArray"=w389:errorcluster[])  [unwired: 8 in, 2 out]
        n176 = for {
          tunnel: w389 -> [w401] mode=indexing
          tunnel: [w393] -> w388 mode=concatenating
          n177 = Unbundle By Name(w401) -> ("source"=w395:string)
          n178 = call <userlib>:"GeneralHandler.vi"("error in (no error)"=w401) -> ("Severity"=w394:string, "Stop"=w398:bool, "Abort"=w399:bool, "Continue"=w400:bool)  [unwired: 7 in]
          n179 = Build Array(w400, w399, w398) -> (w397:bool[])
          n180 = Boolean Array To Number(Boolean array=w397) -> (number=w396:u32)
          n181 = case shown="1" w396 {
            tunnel: w395 -> [_ _ _ _]
            tunnel: w394 -> [_ w402 _ _]
            tunnel: [_ _ w403 w409] -> w393
            frame 0, Default {
              # "No Dialog"
            }
            frame 1 {
              # "Continue"
              n182 = case shown="Default" w402 {
                frame Default {
                  # "Continue operation"
                }
                frame "Log" {
                  # "TODO: if your program\nhas a log file.  Write to \nit here."
                  # "Write to log file"
                }
              }
            }
            frame 2 {
              # "Abort Button Pressed"
              n183 = call "ObtainQueue.vi"() -> ("ErrorArray"=w406:errorcluster[], "QueueRef"=w408:refnum<queue>)  [unwired: 10 in]
              n184 = Flush Queue(queue=w408) -> (error out=w407:errorcluster)  [unwired: 1 in, 2 out]
              n185 = call <userlib>:"AddError.vi"("Severity"="Critical", "Priority"=u8 1, "ErrorArray"=w406, "error in (no error)"=w407) -> ("ErrorArray"=w403:errorcluster[])  [unwired: 6 in, 1 out]
            }
            frame 4 {
              n186 = call "StopEvent.vi"() -> ("ErrorArray"=w409:errorcluster[])  [unwired: 11 in]
            }
          }
        }
      }
      frame Default {
        n187 = xnode "Error Ring"("parameter 0"=w415) -> ("error out"=w414:errorcluster)
        n188 = call <userlib>:"AddError.vi"("Severity"="Inform", "Priority"=u8 5, "ErrorArray"=w412, "error in (no error)"=w414) -> ("ErrorArray"=w413:errorcluster[])  [unwired: 6 in, 1 out]
      }
    }
    n189 = call <extravilib>:"Write.vi"("element"=w71) -> ("channel"=w70:T12)  [unwired: 1 out]
    n190 = call "EnqueError.vi"("ErrorArray"=w75) -> ("ErrorArray 2"=w74:errorcluster[])  [unwired: 10 in]
  }
  n191 = while {
    tunnel: w35 -> [w427]
    shift-right: [w424] -> _
    shift-left: w6 -> [w426]
    stop <- w423 stop-if-true
    # "My Event Handler"
    n192 = event shown="[7] \"rngSync\", \"rngFGen\", \"rngDigitizer\", \"rngAnalysis\", \"rngSensor\": Value Change" {
      selector: w427 -> [w447 _ _ _ _ _ _ _ _ _ _ _ _ _ _ _]
      dyn-events: [w446 _ _ _ _ _ _ _ _ _ _ _ _ _ _ _] -> _
      timeout: _ -> [_ _ _ _ _ _ _ _ _ _ _ _ _ _ _ _]
      tunnel: w426 -> [w454 w466 w482 w483 w505 w509 w513 w529 w571 w607 w612 w617 w622 w645 w670 w677]
      tunnel: [w441 w465 w481 w487 w504 w508 w514 w528 w569 w606 w611 w616 w618 w640 w658 w675] -> w425
      tunnel: [_ _ _ _ _ _ _ _ _ _ TRUE TRUE _ _ _ _] -> w423
      event User Event {
        # "Gets existing bus class\nor creates new"
        # "Remove all buses if any exist"
        n193 = event-data() -> ()  [unwired: 1 in, 1 out]
        n194 = call "GetCntrlRefs.vi"() -> ("CntrlRefs"=w436:T1)  [unwired: 11 in]
        n195 = call "SetGetBus.vi"() -> ("Bus.lvclass"=w438:refnum<class "Bus.lvclass">)  [unwired: 11 in]
        n196 = Unbundle By Name(w436) -> ("btnHideMods"=w435:refnum<vi>)
        n197 = property class="Bus.lvclass"(reference=w438) -> (reference out=w455:refnum<class "Bus.lvclass">, "Accessors:BusNumber"=w456:i32[])  [unwired: 1 in, 1 out]
        n198 = property class="Bool"(reference=w435) -> ("Value"=w434:variant)  [unwired: 1 in, 2 out]
        n199 = for {
          tunnel: w456 -> [w458] mode=indexing
          shift-right: [w459] -> w453
          shift-left: w454 -> [w460]
          shift-right: [w457] -> w452
          shift-left: w455 -> [w461]
          n200 = call "RemoveBus.vi"("BusNumber"=w458, "ErrorIn"=w460, "Bus.lvclass"=w461) -> ("ErrorOut"=w459:errorcluster[], "Bus.lvclass"=w457:refnum<class "Bus.lvclass">)  [unwired: 7 in]
        }
        n201 = call "SetGetModuleList.vi"() -> ("ModuleList"=w437:string[])  [unwired: 11 in]
        n202 = Variant To Data(type=TRUE, Variant=w434) -> (data=w432:bool)  [unwired: 1 in, 1 out]
        n203 = Not(x=w432) -> (.not. x?=w431:bool)
        n204 = call "AddBus.vi"("ShowPanel? (f)"=w431, "BusNumber"=1, "ErrorIn"=w453, "ModuleList"=w437, "Bus.lvclass"=w452) -> ("ErrorOut"=w449:errorcluster[], "UsrEvents"=w448:variant[], "Bus.lvclass"=w450:refnum<class "Bus.lvclass">)  [unwired: 4 in]
        n205 = call "SetGetBus.vi"("Set (f)"=TRUE, "Bus.lvclass"=w450) -> ()  [unwired: 9 in, 1 out]
        n206 = call "BusEvents.vi"("EventArray"=w448, "Error in"=w449, "ModuleList"=w437) -> ("SyncEvts"=w445:T2, "FGenEvts"=w444:T3, "DigitizerEvts"=w443:T4, "AnalysisBroadcastEvents"=w430:T6, "SensorBdcstEvents"=w429:T5, "Error out"=w442:errorcluster[])  [unwired: 16 in, 3 out]
        n207 = To Variant(anything=w437) -> (Variant=w428:variant)
        n208 = register-events(reference=w447, w445, w444, w443, w430, w429) -> (reference out=w446:refnum<event-registration>)  [unwired: 2 in, 1 out]
        n209 = call "Enqueue.vi"("ErrorArray"=w442, "Message Data"=w428, "Message"="InitBus") -> ("ErrorArray"=w441:errorcluster[])  [unwired: 8 in]
      }
      event "btnHideMods": Value Change {
        n210 = event-data() -> ("NewVal"=w475:bool)  [unwired: 1 in]
        n211 = call "SetGetModuleList.vi"() -> ("ModuleList"=w474:string[])  [unwired: 11 in]
        n212 = Select(t="false", s=w475, f="true") -> (s? t:f=w473:string)
        n213 = for {
          tunnel: w474 -> [w479] mode=indexing
          tunnel: w473 -> [w476]
          tunnel: [w478] -> w472 mode=indexing
          n214 = Concatenate Strings("HideModule,", w479, ",", w476) -> (w478:string)
        }
        n215 = call "SetGetBus.vi"() -> ("Bus.lvclass"=w470:refnum<class "Bus.lvclass">)  [unwired: 11 in]
        n216 = property class="Bus.lvclass"(reference=w470) -> ("Accessors:Test"=w469:refnum<class "Test.lvclass">[])  [unwired: 1 in, 2 out]
        n217 = Index Array(array=w469, index=0) -> (element=w467:refnum<class "Test.lvclass">)
        n218 = Build Array (concatenate)(w472, "Stop" ("string")) -> (w464:string[])
        n219 = call "ScriptedStateMachine.vi"("ErrorArray"=w466, "script"=w464, "Test.lvclass"=w467) -> ("ErrorArray"=w465:errorcluster[])  [unwired: 6 in, 2 out]
      }
      event "btnSettings": Value Change {
        n220 = event-data() -> ()  [unwired: 1 in, 1 out]
        n221 = call "Settings.vi"("ErrorArray"=w482) -> ("ErrorArray"=w481:errorcluster[])  [unwired: 10 in]
      }
      event "btnScriptFile": Value Change {
        n222 = event-data() -> ()  [unwired: 1 in, 1 out]
        n223 = call "GetSetConfigClass.vi"() -> ("Ref out"=w495:refnum<class "Config.lvclass">)  [unwired: 11 in]
        n224 = property class="Config.lvclass"(reference=w495) -> ("Accessors:Root Directory"=w494:T11)  [unwired: 1 in, 2 out]
        n225 = Unbundle By Name(w494) -> ("pathRootDir"=w492:path, "ScriptDir"=w493:string)
        n226 = Build Path(base path=w492, name or relative path=w493) -> (appended path=w488:path)
        n227 = call "File Dialog"("start path"=w488) -> ("selected path"=w489:path, "cancelled"=w491:bool, "error out"=w490:errorcluster)  [unwired: 11 in, 1 out]
        n228 = case shown="False" w491 {
          tunnel: w490 -> [w499 w502]
          tunnel: w489 -> [w500 _]
          tunnel: w488 -> [w501 _]
          tunnel: [w496 w502] -> w486
          frame False {
            n229 = call <vilib>:"Compare Two Paths.vi"("error in (no error)"=w499, "Path 2"=w500, "Path 1"=w501) -> ("error out"=w496:errorcluster, "Relative Path from 1 to 2"=w498:path)  [unwired: 5 in, 2 out]
            n230 = Path To String(path=w498) -> (string=w497:string)
            n231 = local write "Test Script"(w497) -> ()
          }
          frame True {
          }
        }
        n232 = call <userlib>:"AddError.vi"("Severity"="Inform", "Priority"=u8 5, "ErrorArray"=w483, "error in (no error)"=w486) -> ("ErrorArray"=w487:errorcluster[])  [unwired: 6 in, 1 out]
      }
      event "btnRunOne": Value Change {
        n233 = event-data() -> ()  [unwired: 1 in, 1 out]
        n234 = call "Enqueue.vi"("ErrorArray"=w505, "Message"="RunOneTest") -> ("ErrorArray"=w504:errorcluster[])  [unwired: 9 in]
      }
      event "btnAbort": Value Change {
        n235 = event-data() -> ()  [unwired: 1 in, 1 out]
        n236 = call "Enqueue.vi"("Priority? (f)"=TRUE, "ErrorArray"=w509, "Message"="Abort") -> ("ErrorArray"=w508:errorcluster[])  [unwired: 8 in]
      }
      event "btnRunScript": Value Change {
        n237 = event-data() -> ()  [unwired: 1 in, 1 out]
        n238 = call "GetSetConfigClass.vi"() -> ("Ref out"=w521:refnum<class "Config.lvclass">)  [unwired: 11 in]
        n239 = property class="Config.lvclass"(reference=w521) -> ("Accessors:Root Directory"=w520:T11)  [unwired: 1 in, 2 out]
        n240 = String To Path(string="Test Script") -> (path=w516:path)
        n241 = Unbundle By Name(w520) -> ("pathRootDir"=w518:path, "ScriptDir"=w519:string)
        n242 = call "RunPython.vi"("PathToScript"=w516, "PathToUserDir"=w518, "ScriptDir"=w519, "keep cmd window open (f)"="chkLeaveScriptWindowOpen") -> ("error out"=w512:errorcluster)  [unwired: 5 in, 1 out]
        n243 = call <userlib>:"AddError.vi"("Severity"="User", "Priority"=u8 3, "ErrorArray"=w513, "error in (no error)"=w512) -> ("ErrorArray"=w514:errorcluster[])  [unwired: 6 in, 1 out]
      }
      event "rngSync", "rngFGen", "rngDigitizer", "rngAnalysis", "rngSensor": Value Change {
        n244 = event-data() -> ("CtlRef"=w533:refnum<vi>)  [unwired: 1 in]
        n245 = call "SetGetBus.vi"() -> ("Bus.lvclass"=w525:refnum<class "Bus.lvclass">)  [unwired: 11 in]
        n246 = property class="Bus.lvclass"(reference=w525) -> (reference out=w523:refnum<class "Bus.lvclass">, "Accessors:Test"=w522:refnum<class "Test.lvclass">[])  [unwired: 1 in, 1 out]
        n247 = property class="Ring (strict)"(reference=w533) -> ("Label.Text"=w532:string, "Value"=w527:u16)  [unwired: 1 in, 2 out]
        n248 = Index Array(array=w522, index=0) -> (element=w524:refnum<class "Test.lvclass">)
        n249 = case shown="Default" w532 {
          selector: w532 -> [_ _ _ _ _ w560]
          tunnel: ["Sync" "FGen" "Digitizer" "Sensor" "Analysis" _] -> w530
          tunnel: [_ _ _ _ _ w561] -> w531
          frame "rngSync" {
          }
          frame "rngFGen" {
          }
          frame "rngDigitizer" {
          }
          frame "rngSensor" {
          }
          frame "rngAnalysis" {
          }
          frame Default {
            n250 = xnode ("Error Ring")("parameter 0"=w560) -> ("error out"=w561:errorcluster)
          }
        }
        n251 = case shown="No Error" w531 {
          selector: w531 -> [_ w551]
          tunnel: w529 -> [w544 w554]
          tunnel: w530 -> [w543 _]
          tunnel: [w548 w550] -> w528
          tunnel: w527 -> [w542 _]
          tunnel: w524 -> [w541 _]
          tunnel: w523 -> [w534 _]
          tunnel: w522 -> [w538 _]
          frame No Error {
            n252 = call "UpdatePluginIndex.vi"("Error"=w544, "Index"=w542, "PluginName"=w543, "Test"=w541) -> ("Error"=w540:errorcluster[], "Test"=w539:refnum<class "Test.lvclass">)  [unwired: 6 in]
            n253 = Replace Array Subset(array=w538, new element=w539) -> (w537:refnum<class "Test.lvclass">[])  [unwired: 1 in]
            n254 = property class="Bus.lvclass"(reference=w534, "Accessors:Test"=w537) -> (reference out=w536:refnum<class "Bus.lvclass">)  [unwired: 1 in, 1 out]
            n255 = Concatenate Strings("LoadPlugin,", w543) -> (w545:string)
            n256 = Build Array(w545, "Stop") -> (w547:string[])
            n257 = call "ScriptedStateMachine.vi"("ErrorArray"=w540, "script"=w547, "Test.lvclass"=w539) -> ("ErrorArray"=w548:errorcluster[])  [unwired: 6 in, 2 out]
            n258 = call "SetGetBus.vi"("Set (f)"=TRUE, "Bus.lvclass"=w536) -> ()  [unwired: 9 in, 1 out]
          }
          frame Error {
            n259 = call <userlib>:"AddError.vi"("Severity"="Abort", "Priority"=u8 3, "ErrorArray"=w554, "error in (no error)"=w551) -> ("ErrorArray"=w550:errorcluster[])  [unwired: 6 in, 1 out]
          }
        }
      }
      event "btnSyncPref", "btnFGenPref", "btnDigitizerPref", "btnAnalysisPref", "btnSensorPref": Value Change {
        n260 = event-data() -> ("CtlRef"=w574:refnum<vi>)  [unwired: 1 in]
        n261 = property class="Bool"(reference=w574) -> ("Label.Text"=w573:string)  [unwired: 1 in, 2 out]
        n262 = case shown="\"btnSensorPref\"" w573 {
          selector: w573 -> [_ _ _ _ _ w596]
          tunnel: ["Sync" "FGen" "Digitizer" "Sensor" "Analysis" _] -> w570
          tunnel: [_ _ _ _ _ w597] -> w572
          frame "btnSyncPref" {
          }
          frame "btnFGenPref" {
          }
          frame "btnDigitizerPref" {
          }
          frame "btnSensorPref" {
          }
          frame "btnAnalysisPref" {
          }
          frame Default {
            n263 = xnode ("Error Ring")("parameter 0"=w596) -> ("error out"=w597:errorcluster)
          }
        }
        n264 = case shown="Error" w572 {
          selector: w572 -> [_ w587]
          tunnel: w571 -> [w584 w590]
          tunnel: w570 -> [w576 _]
          tunnel: [w583 w586] -> w569
          frame No Error {
            n265 = call "SetGetBus.vi"() -> ("Bus.lvclass"=w580:refnum<class "Bus.lvclass">)  [unwired: 11 in]
            n266 = property class="Bus.lvclass"(reference=w580) -> ("Accessors:Test"=w581:refnum<class "Test.lvclass">[])  [unwired: 1 in, 2 out]
            n267 = Concatenate Strings("PrefDlgRequest,", w576) -> (w575:string)
            n268 = Index Array(array=w581, index=0) -> (element=w579:refnum<class "Test.lvclass">)
            n269 = Build Array(w575, "Stop") -> (w578:string[])
            n270 = call "ScriptedStateMachine.vi"("ErrorArray"=w584, "script"=w578, "Test.lvclass"=w579) -> ("ErrorArray"=w583:errorcluster[])  [unwired: 6 in, 2 out]
          }
          frame Error {
            n271 = call <userlib>:"AddError.vi"("Severity"="Inform", "Priority"=u8 4, "ErrorArray"=w590, "error in (no error)"=w587) -> ("ErrorArray"=w586:errorcluster[])  [unwired: 6 in, 1 out]
          }
        }
      }
      event "btnVisualize": Value Change {
        n272 = event-data() -> ()  [unwired: 1 in, 1 out]
        n273 = call "Enqueue.vi"("ErrorArray"=w607, "Message"="Visualize") -> ("ErrorArray"=w606:errorcluster[])  [unwired: 9 in]
      }
      event "btnStop": Value Change {
        n274 = event-data() -> ()  [unwired: 1 in, 1 out]
        n275 = call "Enqueue.vi"("Priority (F)"=TRUE, "ErrorArray"=w612, "Message"="Stop") -> ("ErrorArray"=w611:errorcluster[])  [unwired: 8 in]
      }
      event User Event {
        n276 = event-data() -> ()  [unwired: 1 in, 1 out]
        n277 = call "Enqueue.vi"("Priority (F)"=TRUE, "ErrorArray"=w617, "Message"="Stop") -> ("ErrorArray"=w616:errorcluster[])  [unwired: 8 in]
      }
      event User Event {
        n278 = event-data() -> ("Data"=w638:variant)  [unwired: 1 in]
        n279 = Get Date/Time In Seconds() -> (seconds since 1Jan1904=w633:timestamp)
        n280 = Variant To Data(type=T14 {"Init?"=FALSE, "ModuleAdmin"=refnum} ("clDidInit"), Variant=w638) -> (data=w636:T14, error out=w626:errorcluster)  [unwired: 1 in]
        n281 = Get Date/Time String(date format (0)=enum16{"short", "long", "abbreviated"}."short", seconds (now)=w633, want seconds? (F)=TRUE) -> (time string=w630:string)  [unwired: 1 out]
        n282 = Unbundle By Name(w636) -> ("ModuleAdmin"=w635:refnum<class "ModuleAdmin.lvclass">)
        n283 = property class="ModuleAdmin.lvclass"(reference=w635) -> ("Accessors:ModuleName"=w629:string, "Accessors:Module ID"=w628:i32)  [unwired: 1 in, 2 out]
        n284 = Format Into String(format string="%s: %s: %d %s \\r", error in=w626, w630, w629, w628, "Did Init" ("input 4")) -> (resulting string=w625:string, error out=w621:errorcluster)  [unwired: 1 in]
        n285 = call <userlib>:"AddError.vi"("Severity"="Inform", "Priority"=u8 4, "ErrorArray"=w622, "error in (no error)"=w621) -> ("ErrorArray"=w623:errorcluster[])  [unwired: 6 in, 1 out]
        n286 = call "AddLogMsg.vi"("LogLevel"=eLogLvl."Normal", "Error"=w623, "LogMessage"=w625) -> ("Error"=w618:errorcluster[])  [unwired: 8 in]
      }
      event User Event {
        n287 = event-data() -> ("Data"=w655:variant)  [unwired: 1 in]
        n288 = Get Date/Time In Seconds() -> (seconds since 1Jan1904=w653:timestamp)
        n289 = Variant To Data(type="", Variant=w655) -> (data=w648:string, error out=w647:errorcluster)  [unwired: 1 in]
        n290 = Get Date/Time String(date format (0)=enum16{"short", "long", "abbreviated"}."short", seconds (now)=w653, want seconds? (F)=TRUE) -> (time string=w649:string)  [unwired: 1 out]
        n291 = Format Into String(format string="%s: %s \\r", error in=w647, w649, w648) -> (resulting string=w646:string, error out=w643:errorcluster)  [unwired: 1 in]
        n292 = call <userlib>:"AddError.vi"("Severity"="Inform", "Priority"=u8 4, "ErrorArray"=w645, "error in (no error)"=w643) -> ("ErrorArray"=w644:errorcluster[])  [unwired: 6 in, 1 out]
        n293 = call "AddLogMsg.vi"("LogLevel"=eLogLvl."Normal", "Error"=w644, "LogMessage"=w646) -> ("Error"=w640:errorcluster[])  [unwired: 8 in]
      }
      event User Event {
        n294 = event-data() -> ("ModuleID"=w662:i32, "Data"=w674:variant)  [unwired: 1 in]
        n295 = Get Date/Time In Seconds() -> (seconds since 1Jan1904=w666:timestamp)
        n296 = Variant To Data(type=errorcluster {"status"=FALSE, "code"=0, "source"=""} ("error constant"), Variant=w674) -> (data=w671:errorcluster, error out=w672:errorcluster)  [unwired: 1 in]
        n297 = Get Date/Time String(date format (0)=enum16{"short", "long", "abbreviated"}."short", seconds (now)=w666, want seconds? (F)=TRUE) -> (time string=w663:string)  [unwired: 1 out]
        n298 = Unbundle By Name(w671) -> ("source"=w661:string)
        n299 = Merge Errors(w671, w672) -> (w669:errorcluster)
        n300 = call <userlib>:"AddError.vi"("Severity"="UserOption", "Priority"=u8 2, "ErrorArray"=w670, "error in (no error)"=w669) -> ("ErrorArray"=w660:errorcluster[])  [unwired: 6 in, 1 out]
        n301 = Format Into String(format string="%s: Module %d:  %s \\r", w663, w662, w661) -> (resulting string=w659:string)  [unwired: 2 in, 1 out]
        n302 = call "AddLogMsg.vi"("LogLevel"=eLogLvl."Normal", "Error"=w660, "LogMessage"=w659) -> ("Error"=w658:errorcluster[])  [unwired: 8 in]
      }
      event User Event {
        n303 = event-data() -> ("Data"=w680:variant)  [unwired: 1 in]
        n304 = Variant To Data(type=TRUE, Variant=w680) -> (data=→"Locked":bool, error out=w676:errorcluster)  [unwired: 1 in]
        n305 = call <userlib>:"AddError.vi"("ErrorArray"=w677, "error in (no error)"=w676) -> ("ErrorArray"=w675:errorcluster[])  [unwired: 8 in, 1 out]
      }
    }
    n306 = call "EnqueError.vi"("ErrorArray"=w425) -> ("ErrorArray 2"=w424:errorcluster[])  [unwired: 10 in]
  }
  n307 = call "ObtainTCPSocket.vi"("ErrorArray"=w6, "timeout"=25) -> ("ErrorArray"=w4:errorcluster[])  [unwired: 8 in, 1 out]
  n308 = while {
    shift-right: [w682] -> w3
    shift-left: w4 -> [w686]
    tunnel: w1 -> [w681]
    stop <- w687 stop-if-true
    n309 = call <extravilib>:"Read.vi"("channel"=w681) -> ("element"=w687:bool)  [unwired: 1 in, 1 out]
    n310 = call "Listener.vi"("ErrorArray"=w686) -> ("ErrorArray"=w685:errorcluster[], "Accepted?"=w684:bool)  [unwired: 9 in]
    n311 = case shown="True" w684 {
      tunnel: w685 -> [w689 w692]
      tunnel: [w689 w690] -> w683
      tunnel: w681 -> [_ w691]
      frame False {
        n312 = Wait (ms)(milliseconds to wait=u32 10) -> ()  [unwired: 1 out]
      }
      frame True {
        n313 = while {
          tunnel: w692 -> [w703]
          tunnel: w691 -> [w698]
          tunnel: [w697] -> w690
          stop <- w695 stop-if-true
          n314 = call <extravilib>:"Read.vi"("channel"=w698) -> ("element"=w694:bool)  [unwired: 1 in, 1 out]
          n315 = call "Receiver.vi"("ErrorArray"=w703) -> ("ErrorArray"=w699:errorcluster[], "XMLData"=w700:string, "Command"=w701:string, "error out"=w693:errorcluster, "bytes_read"=w702:i32)  [unwired: 6 in]
          n316 = Or(x=w694, y=w693) -> (x .or. y?=w695:bool)
          n317 = case shown="1, Default" w702 {
            tunnel: w701 -> [_ w706]
            tunnel: w700 -> [_ w707]
            tunnel: w699 -> [w704 w709]
            tunnel: [w704 w705] -> w696
            frame 0 {
            }
            frame 1, Default {
              n318 = To Variant(anything=w707) -> (Variant=w708:variant)
              n319 = call "Enqueue.vi"("ErrorArray"=w709, "Message Data"=w708, "Message"=w706) -> ("ErrorArray"=w705:errorcluster[])  [unwired: 8 in]
            }
          }
          n320 = call "EnqueError.vi"("ErrorArray"=w696) -> ("ErrorArray 2"=w697:errorcluster[])  [unwired: 10 in]
        }
      }
    }
    n321 = call "EnqueError.vi"("ErrorArray"=w683) -> ("ErrorArray 2"=w682:errorcluster[])  [unwired: 10 in]
  }
  n322 = call "Disconnect.vi"("ErrorArray"=w3) -> ()  [unwired: 10 in, 1 out]
